vi "Order of Transformations.vi"() -> ()   [LabVIEW 2016]
doc: "This VI demonstrates how the order in which you apply transformations to an object in a 3D scene affects the object's position and orientation within the scene. \n\n<b>Rotate then Translate:</b>\nIf you apply a rotation to an object as the first transformation, the object rotates around its parent's axis, which exists in spatially the same place as the object's own axis. Regardless of what transformations follow the rotation, the object appears to rotate around its own axis. If you apply a translation after the rotation, the object appears offset from its parent and still spinning around its own axis.\n\n<b>Translate then Rotate:</b>\nIf you apply a translation to an object as the first transformation, the object still appears offset from its parent. However, if you then apply a rotation to the object, the object rotates around its parent by the angle you specify with the Translate Object VI."
uses:
  <vilib>/picture/3D Picture Control/Object/Create Object (drawable).vi
  <vilib>/picture/3D Picture Control/Object/Add Object (reference).vi
  <vilib>/picture/3D Picture Control/NI_3D Picture Control.lvlib
panel:
  in  "Child (Yellow Cone)":u16(ring) items=["No Transform", "Rotate then Translate", "Translate then Rotate"]
  in  "Stop":bool
  in  "Parent (Red Box)":u16(ring) items=["No Transform", "Rotate then Translate", "Translate then Rotate"]
  out "3D Picture":refnum<vi>(3d-picture)
  # "Overview: This VI demonstrates how to construct a hierarchy of objects within a 3D Picture, and how the order in which you apply transformations to an object affects the object's position and orientation.\nInstructions:\n1. Run the VI.\n2. Change the values of the Parent and Child rings to change the order in which transformations apply to each object.\n3. Click Stop to stop the VI."
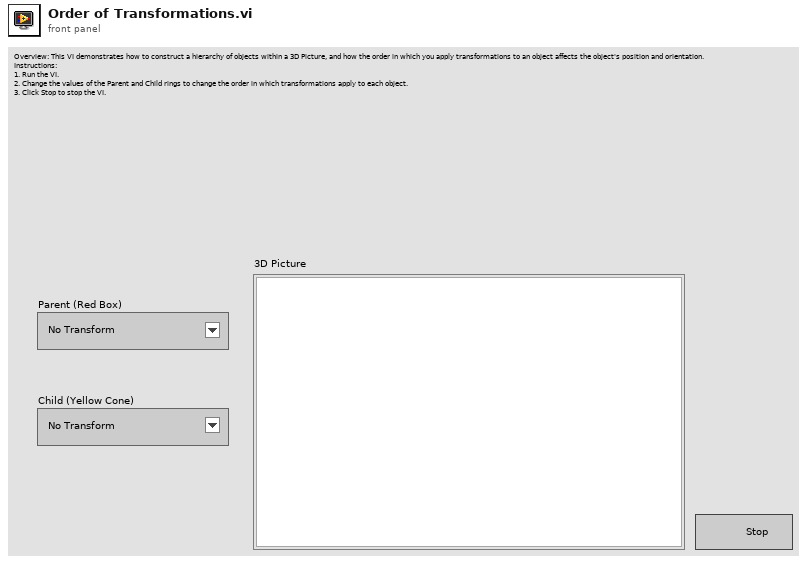
[diagram p1: front panel]
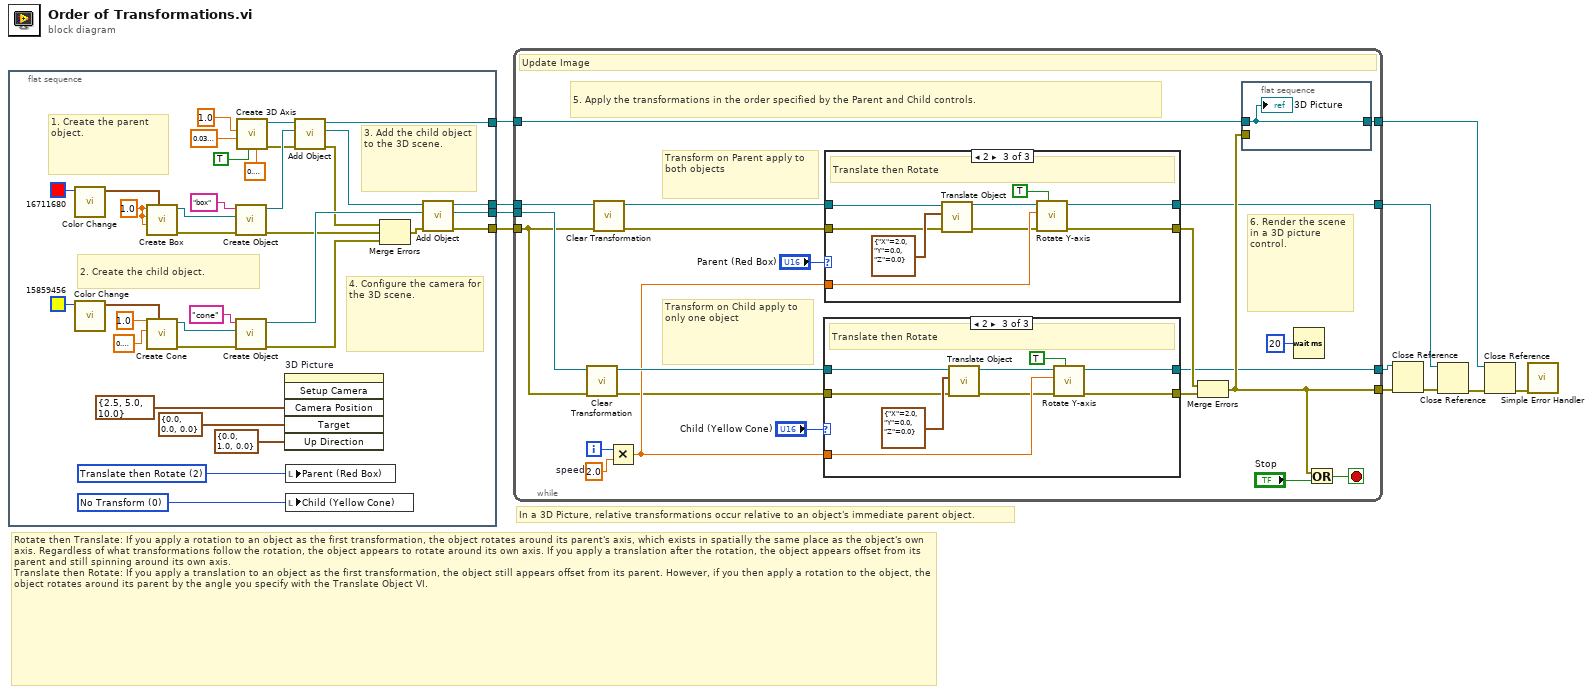
[diagram p0: block diagram]
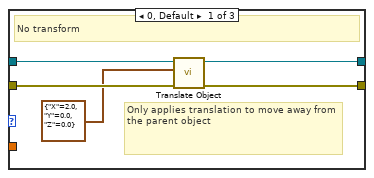
[diagram p2: hidden frame]
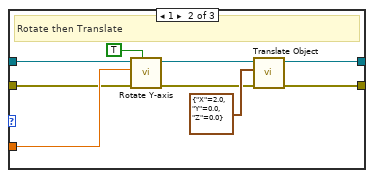
[diagram p3: hidden frame]
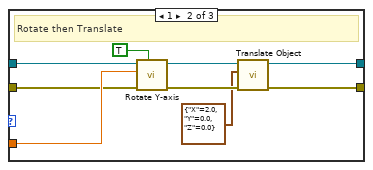
[diagram p5: hidden frame]
diagram:
  # "Rotate then Translate: If you apply a rotation to an object as the first transformation, the object rotates around its parent's axis, which exists in spatially the same place as the object's own axis. Regardless of what transformations follow the rotation, the object appears to rotate around its own axis. If you apply a translation after the rotation, the object appears offset from its parent and still spinning around its own axis.\nTranslate then Rotate: If you apply a translation to an object as the first transformation, the object still appears offset from its parent. However, if you then apply a rotation to the object, the object rotates around its parent by the angle you specify with the Translate Object VI."
  # "In a 3D Picture, relative transformations occur relative to an object's immediate parent object."
  n1 = flat-sequence {
    tunnel: [w33] -> w11
    tunnel: [w34] -> w10
    tunnel: [w26] -> w9
    tunnel: [w20] -> w8
    frame #0 {
      w15 = sgl 1.0 ("Length X")
      w38 = u16 0 items=["No Transform", "Rotate then Translate", "Translate then Rotate"] ("Child (Yellow)")
      w39 = u16 2 items=["No Transform", "Rotate then Translate", "Translate then Rotate"] ("Parent (Red)")
      # "2. Create the child object."
      # "4. Configure the camera for the 3D scene."
      # "3. Add the child object to the 3D scene."
      # "1. Create the parent object."
      n2 = call <vilib>:"Color Change.vi"("Color"=u32 16711680) -> ("RGBA"=w43:cluster{"R":sgl, "G":sgl, "B":sgl, "A":sgl})  [unwired: 10 in]
      n3 = call <vilib>:"Color Change.vi"("Color"=u32 15859456) -> ("RGBA"=w46:cluster{"R":sgl, "G":sgl, "B":sgl, "A":sgl})  [unwired: 10 in]
      n4 = call <vilib>:"Create Box.vi"("Color"=w43, "Length Z"=w15, "Length Y"=w15, "Length X"=w15) -> ("error out"=w32:errorcluster, "New Box Refnum"=w37:refnum<vi>)  [unwired: 6 in]
      n5 = call <vilib>:"Create Cone.vi"("Color"=w46, "Radius"=sgl 0.6, "Height"=sgl 1.0) -> ("error out"=w31:errorcluster, "New Cone Refnum"=w36:refnum<vi>)  [unwired: 7 in]
      n6 = call-poly <vilib>:"Create Object.vi"("error in (no error)"=w32, "Geometry"=w37, "Name"="box") -> ("error out"=w29:errorcluster, "Scene:New Object"=w23:refnum<vi>)  [unwired: 7 in]
      n7 = call-poly <vilib>:"Create Object.vi"("error in (no error)"=w31, "Geometry"=w36, "Name"="cone") -> ("error out"=w28:errorcluster, "Scene:New Object"=w35:refnum<vi>)  [unwired: 7 in]
      n8 = call <vilib>:"Create 3D Axis.vi"("Character Size"=sgl 0.4, "Axis label?"=TRUE, "Radius"=sgl 0.04, "Length"=sgl 1.0) -> ("error out"=w17:errorcluster, "New Object Refnum"=w21:refnum<vi>)  [unwired: 6 in]
      n9 = invoke on="3D Picture" class="SceneGraphDisp (strict)" method="Setup Camera"("Camera Position"=cluster{"X":sgl, "Y":sgl, "Z":sgl} {"X"=2.5, "Y"=5.0, "Z"=10.0}, "Target"=cluster{"X":sgl, "Y":sgl, "Z":sgl} {"X"=0.0, "Y"=0.0, "Z"=0.0}, "Up Direction"=cluster{"X":sgl, "Y":sgl, "Z":sgl} {"X"=0.0, "Y"=1.0, "Z"=0.0}) -> ()  [unwired: 3 in, 6 out]
      n10 = local write "Parent (Red Box)"(w39) -> ()
      n11 = local write "Child (Yellow Cone)"(w38) -> ()
      n12 = call-poly <vilib>:"Add Object.vi"("error in (no error)"=w17, "New Object In"=w23, "Scene Object In"=w21) -> ("error out"=w16:errorcluster, "New Object Out"=w22:refnum<vi>, "Scene Object Out"=w20:refnum<vi>)  [unwired: 6 in]
      n13 = Merge Errors(w16, w29, w28) -> (w27:errorcluster)
      n14 = call-poly <vilib>:"Add Object.vi"("error in (no error)"=w27, "New Object In"=w35, "Scene Object In"=w22) -> ("error out"=w26:errorcluster, "New Object Out"=w34:refnum<vi>, "Scene Object Out"=w33:refnum<vi>)  [unwired: 6 in]
    }
  }
  n15 = while {
    tunnel: w11 -> [w68]
    tunnel: w10 -> [w67]
    tunnel: w9 -> [w59]
    tunnel: [w50] -> w6
    tunnel: w8 -> [w54]
    tunnel: [w49] -> w7
    tunnel: [w48] -> w5
    tunnel: [w47] -> w3
    i -> [w53]
    stop <- w55 stop-if-true
    w62 = 2.0  # speed
    # "6. Render the scene in a 3D picture control."
    # "Transform on Child apply to only one object"
    # "Transform on Parent apply to both objects"
    # "5. Apply the transformations in the order specified by the Parent and Child controls."
    # "Update Image"
    n16 = call <vilib>:"Clear Transformation.vi"("error in (no error)"=w59, "Object Refnum In"=w67) -> ("error out"=w57:errorcluster, "Object Refnum Out"=w64:refnum<vi>)  [unwired: 8 in]
    n17 = call <vilib>:"Clear Transformation.vi"("error in (no error)"=w59, "Object Refnum In"=w68) -> ("error out"=w58:errorcluster, "Object Refnum Out"=w65:refnum<vi>)  [unwired: 8 in]
    n18 = Multiply(x=w53, y=w62) -> (x*y=w63:dbl)
    n19 = case shown="2" "Child (Yellow Cone)" {
      tunnel: w64 -> [w74 w83 w92]
      tunnel: w63 -> [_ w82 w90]
      tunnel: [w73 w80 w89] -> w48
      tunnel: w57 -> [w72 w79 w87]
      tunnel: [w71 w76 w85] -> w56
      frame 0, Default {
        # "Only applies translation to move away from the parent object"
        # "No transform"
        n20 = call <vilib>:"Translate Object.vi"("error in (no error)"=w72, "Translation"=cluster{"X":sgl, "Y":sgl, "Z":sgl} {"X"=2.0, "Y"=0.0, "Z"=0.0}, "Scene.Object In"=w74) -> ("error out"=w71:errorcluster, "Scene.Object Out"=w73:refnum<vi>)  [unwired: 7 in]
      }
      frame 1 {
        # "Rotate then Translate"
        n21 = call <vilib>:"Rotate Y-axis.vi"("Relative?"=TRUE, "error in (no error)"=w79, "angle"=w82, "Scene Object In"=w83) -> ("error out"=w77:errorcluster, "Scene Object Out"=w81:refnum<vi>)  [unwired: 6 in]
        n22 = call <vilib>:"Translate Object.vi"("error in (no error)"=w77, "Translation"=cluster{"X":sgl, "Y":sgl, "Z":sgl} {"X"=2.0, "Y"=0.0, "Z"=0.0}, "Scene.Object In"=w81) -> ("error out"=w76:errorcluster, "Scene.Object Out"=w80:refnum<vi>)  [unwired: 7 in]
      }
      frame 2 {
        # "Translate then Rotate"
        n23 = call <vilib>:"Translate Object.vi"("error in (no error)"=w87, "Translation"=cluster{"X":sgl, "Y":sgl, "Z":sgl} {"X"=2.0, "Y"=0.0, "Z"=0.0}, "Scene.Object In"=w92) -> ("error out"=w86:errorcluster, "Scene.Object Out"=w91:refnum<vi>)  [unwired: 7 in]
        n24 = call <vilib>:"Rotate Y-axis.vi"("Relative?"=TRUE, "error in (no error)"=w86, "angle"=w90, "Scene Object In"=w91) -> ("error out"=w85:errorcluster, "Scene Object Out"=w89:refnum<vi>)  [unwired: 6 in]
      }
    }
    n25 = case shown="2" "Parent (Red Box)" {
      tunnel: w65 -> [w94 w103 w112]
      tunnel: w63 -> [_ w100 w109]
      tunnel: [w94 w101 w108] -> w47
      tunnel: w58 -> [w93 w99 w107]
      tunnel: [w93 w97 w105] -> w51
      frame 0, Default {
        # "No transform"
      }
      frame 1 {
        # "Rotate then Translate"
        n26 = call <vilib>:"Rotate Y-axis.vi"("Relative?"=TRUE, "error in (no error)"=w99, "angle"=w100, "Scene Object In"=w103) -> ("error out"=w98:errorcluster, "Scene Object Out"=w102:refnum<vi>)  [unwired: 6 in]
        n27 = call <vilib>:"Translate Object.vi"("error in (no error)"=w98, "Translation"=cluster{"X":sgl, "Y":sgl, "Z":sgl} {"X"=2.0, "Y"=0.0, "Z"=0.0}, "Scene.Object In"=w102) -> ("error out"=w97:errorcluster, "Scene.Object Out"=w101:refnum<vi>)  [unwired: 7 in]
      }
      frame 2 {
        # "Translate then Rotate"
        n28 = call <vilib>:"Translate Object.vi"("error in (no error)"=w107, "Translation"=cluster{"X":sgl, "Y":sgl, "Z":sgl} {"X"=2.0, "Y"=0.0, "Z"=0.0}, "Scene.Object In"=w112) -> ("error out"=w106:errorcluster, "Scene.Object Out"=w110:refnum<vi>)  [unwired: 7 in]
        n29 = call <vilib>:"Rotate Y-axis.vi"("Relative?"=TRUE, "error in (no error)"=w106, "angle"=w109, "Scene Object In"=w110) -> ("error out"=w105:errorcluster, "Scene Object Out"=w108:refnum<vi>)  [unwired: 6 in]
      }
    }
    n30 = Merge Errors(w51, w56) -> (w50:errorcluster)
    n31 = flat-sequence {
      tunnel: w54 -> [w69]
      tunnel: w50 -> [_]
      tunnel: [w69] -> w49
      frame #0 {
        "3D Picture" <- w69
      }
    }
    n32 = Wait (ms)(milliseconds to wait=u32 20) -> ()  [unwired: 1 out]
    n33 = Or(x=w50, y="Stop") -> (x .or. y?=w55:bool)
  }
  n34 = Close Reference(reference=w5, error in (no error)=w6) -> (error out=w4:errorcluster)
  n35 = Close Reference(reference=w3, error in (no error)=w4) -> (error out=w2:errorcluster)
  n36 = Close Reference(reference=w7, error in (no error)=w2) -> (error out=w1:errorcluster)
  n37 = call <vilib>:"Simple Error Handler.vi"("error in (no error)"=w1) -> ()  [unwired: 4 in, 5 out]
